vi "Filter Gain Array.vi"(8 "error in (no error)":errorcluster, 11 "Gain Ring Reference":refnum<vi>) -> (0 "error out":errorcluster)   [LabVIEW 2017]
doc: "Filters 0 gain values from the gain array."
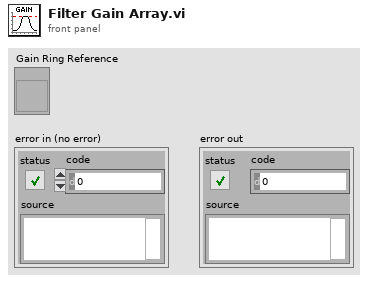
[diagram p1: front panel]
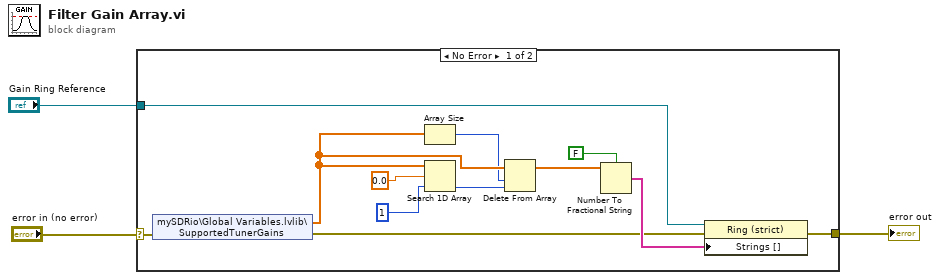
[diagram p0: block diagram]
diagram:
  n1 = case shown="No Error" "error in (no error)" {
    selector: "error in (no error)" -> [w4 w16]
    tunnel: [w15 w16] -> w3
    tunnel: "Gain Ring Reference" -> [w12 _]
    frame No Error {
      n2 = shared-variable "mySDRio\\Global Variables.lvlib\\SupportedTunerGains"(error in=w4) -> (w6:dbl[], error out=w7:errorcluster)
      n3 = Array Size(array=w6) -> (size(s)=w5:i32)
      n4 = Search 1D Array(1D array=w6, element=0.0, start index (0)=1) -> (index of element=w9:i32)
      n5 = Delete From Array(array=w6, length=w5, index=w9) -> (array with subset deleted=w8:dbl[])  [unwired: 1 out]
      n6 = Number To Fractional String(use system decimal point (T)=FALSE, number=w8) -> (F-format string=w14:string[])  [unwired: 2 in]
      n7 = property on="Property Node" class="Ring (strict)"(reference=w12, error in=w7, "Strings []"=w14) -> (error out=w15:errorcluster)  [unwired: 1 out]
    }
    frame Error {
    }
  }
  "error out" <- w3
